vi "Pressure_control_TEMP.vi"(7 "Run Sequence":bool, 8 "user sequence, present (s) in, current step in, seq time in":T6, 9 "pressure parameters in":T1={"valve % open"=100.0, "Desired pressure"=0.0, "set Vapor sccm"=0.0, "set Gas sccm"=0.0, "Valve mode"=enum."% Open", "Pressure Mode"=enum."Abs. pressure", "analyte partial pressure"=100.0, "Turbo pump\nauto on"=TRUE} caption="Set pressure parameters" {"analyte partial pressure" min=0.0 max=100.0 step=5.0; "set Gas sccm" min=0 max=200 step=5; "set Vapor sccm" min=0 max=200 step=5; "Desired pressure" min=0.0 max=760.0 step=5.0; "valve % open" min=0.0 max=100.0 step=5.0 format="%#_2f"}, 10 "set temp":dbl, 11 "pressure control on? / DAQ IDs/errors in":T5) -> (0 "current step # out, shift register time out, seq button on?":T3, 1 "sequence over? USE THIS TO REINITIALIZE RUN SEQUENCE BUTTON SO PROGRAM ENDS":bool, 2 "save press/RH/gasflow/vaporflow - read valve position/pressure/vaporflow/gasflow":T2, 3 "pressure control on out, DAQ IDs/errors out":T4, 4 "sequence end date/time string":string, 5 "Temp setpoint":dbl)   [LabVIEW 2014]
uses:
  <vilib>/DAQmx/read.llb/DAQmx Read (Analog 1D DBL NChan 1Samp).vi
  <vilib>/DAQmx/write.llb/DAQmx Write (Analog 1D DBL NChan 1Samp).vi
  <vilib>/DAQmx/write.llb/DAQmx Write (Digital Bool 1Line 1Point).vi
panel:
  # "100%"
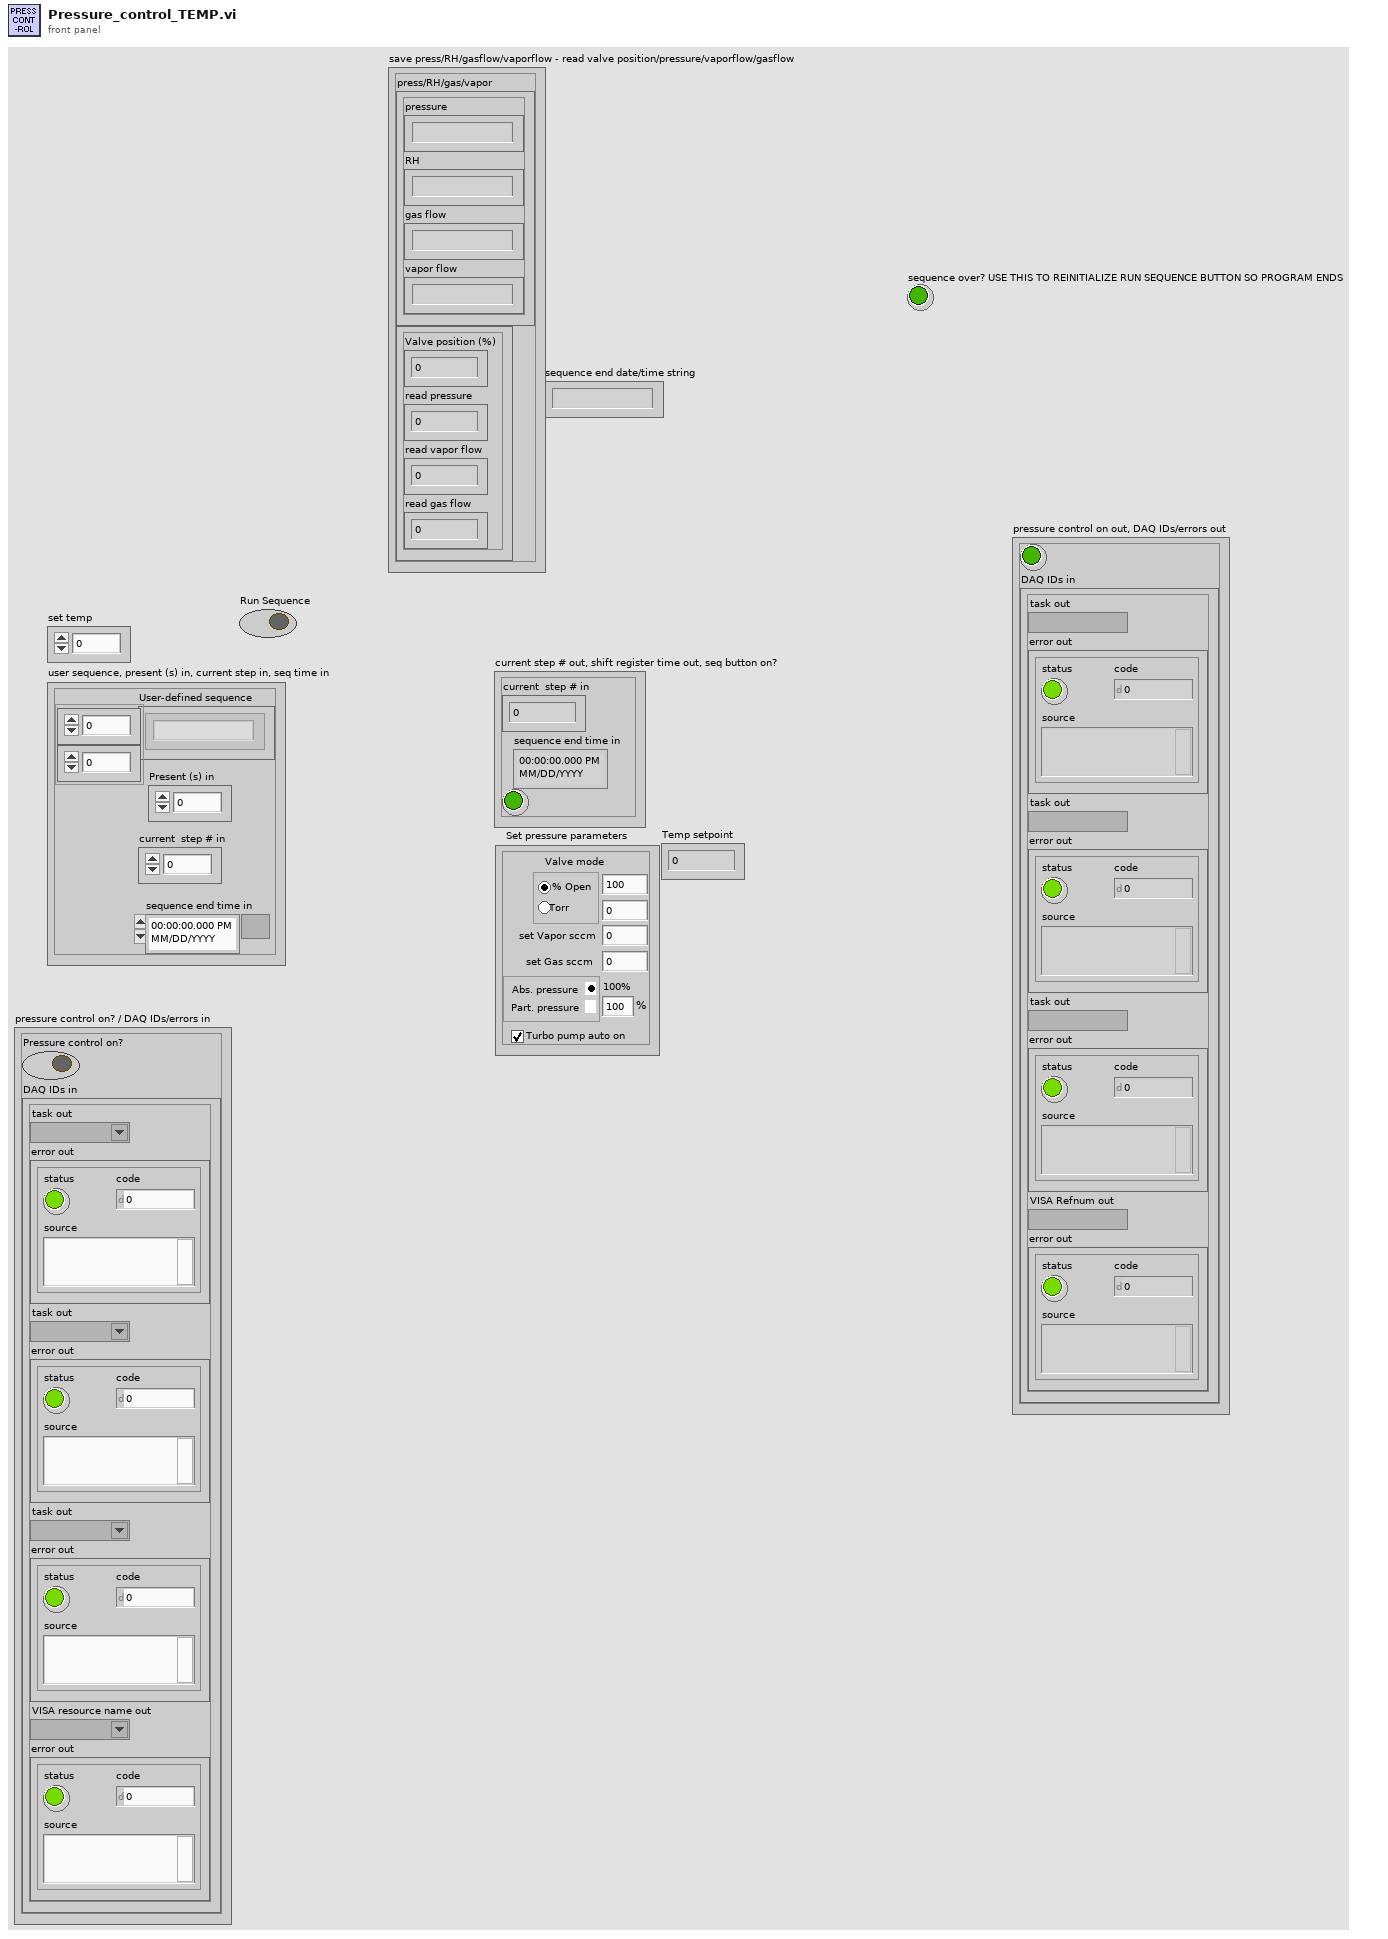
[diagram p1: front panel]
types:
  T1 = cluster{"valve % open":dbl, "Desired pressure":dbl, "set Vapor sccm":sgl, "set Gas sccm":sgl, "Valve mode":enum32{"% Open", "Torr "}, "Pressure Mode":enum32{"Abs. pressure", " Part. pressure"}, "analyte partial pressure":dbl, "Turbo pump\nauto on":bool}
  T2 = cluster{"press/RH/gas/vapor":cluster{"pressure":string, "RH":string, "gas flow":string, "vapor flow":string}, "Cluster":cluster{"Valve position (%)":dbl, "read pressure":dbl, "read vapor flow":dbl, "read gas flow":dbl}}
  T3 = cluster{"current  step # in":i32, "sequence end time in":timestamp, "Boolean":bool}
  T4 = cluster{"Boolean":bool, "DAQ IDs in":cluster{"task out":refnum<k21>, "error out":errorcluster, "task out":refnum<k21>, "error out":errorcluster, "task out":refnum<k21>, "error out":errorcluster, "VISA Refnum out":refnum<visa-resource-name>, "error out":errorcluster}}
  T5 = cluster{"Pressure control on?":bool, "DAQ IDs in":cluster{"task out":refnum<k21>, "error out":errorcluster, "task out":refnum<k21>, "error out":errorcluster, "task out":refnum<k21>, "error out":errorcluster, "VISA resource name out":refnum<visa-resource-name>, "error out":errorcluster}}
  T6 = cluster{"User-defined sequence":string[][], "Present (s) in":dbl, "current  step # in":i32, "sequence end time in":timestamp}
  T7 = cluster{"task out":refnum<k21>, "error out":errorcluster, "task out":refnum<k21>, "error out":errorcluster, "task out":refnum<k21>, "error out":errorcluster, "VISA resource name out":refnum<visa-resource-name>, "error out":errorcluster}
  T8 = cluster{"Valve position (%)":dbl, "pressure":dbl, "vapor flow":dbl, "gas flow":dbl}
  T9 = cluster{"pressure":string, "RH":string, "gas flow":string, "vapor flow":string}
  T10 = cluster{"String":dbl, "String":dbl, "Pressure Control":u32}
  T11 = cluster{"Valve position (%)":dbl, "read pressure":dbl, "read vapor flow":dbl, "read gas flow":dbl}
  T12 = cluster{"task out":refnum<k21>, "error out":errorcluster, "task out":refnum<k21>, "error out":errorcluster, "task out":refnum<k21>, "error out":errorcluster, "VISA Refnum out":refnum<visa-resource-name>, "error out":errorcluster}
  T13 = cluster{"press/RH/gas/vapor":cluster{"pressure":string, "RH":string, "gas flow":string, "vapor flow":string}, cluster{"Valve position (%)":dbl, "read pressure":dbl, "read vapor flow":dbl, "read gas flow":dbl}}
  T14 = cluster{"current  step # in":i32, "sequence end time in":timestamp, bool}
  T15 = cluster{bool, "DAQ IDs in":cluster{"task out":refnum<k21>, "error out":errorcluster, "task out":refnum<k21>, "error out":errorcluster, "task out":refnum<k21>, "error out":errorcluster, "VISA Refnum out":refnum<visa-resource-name>, "error out":errorcluster}}
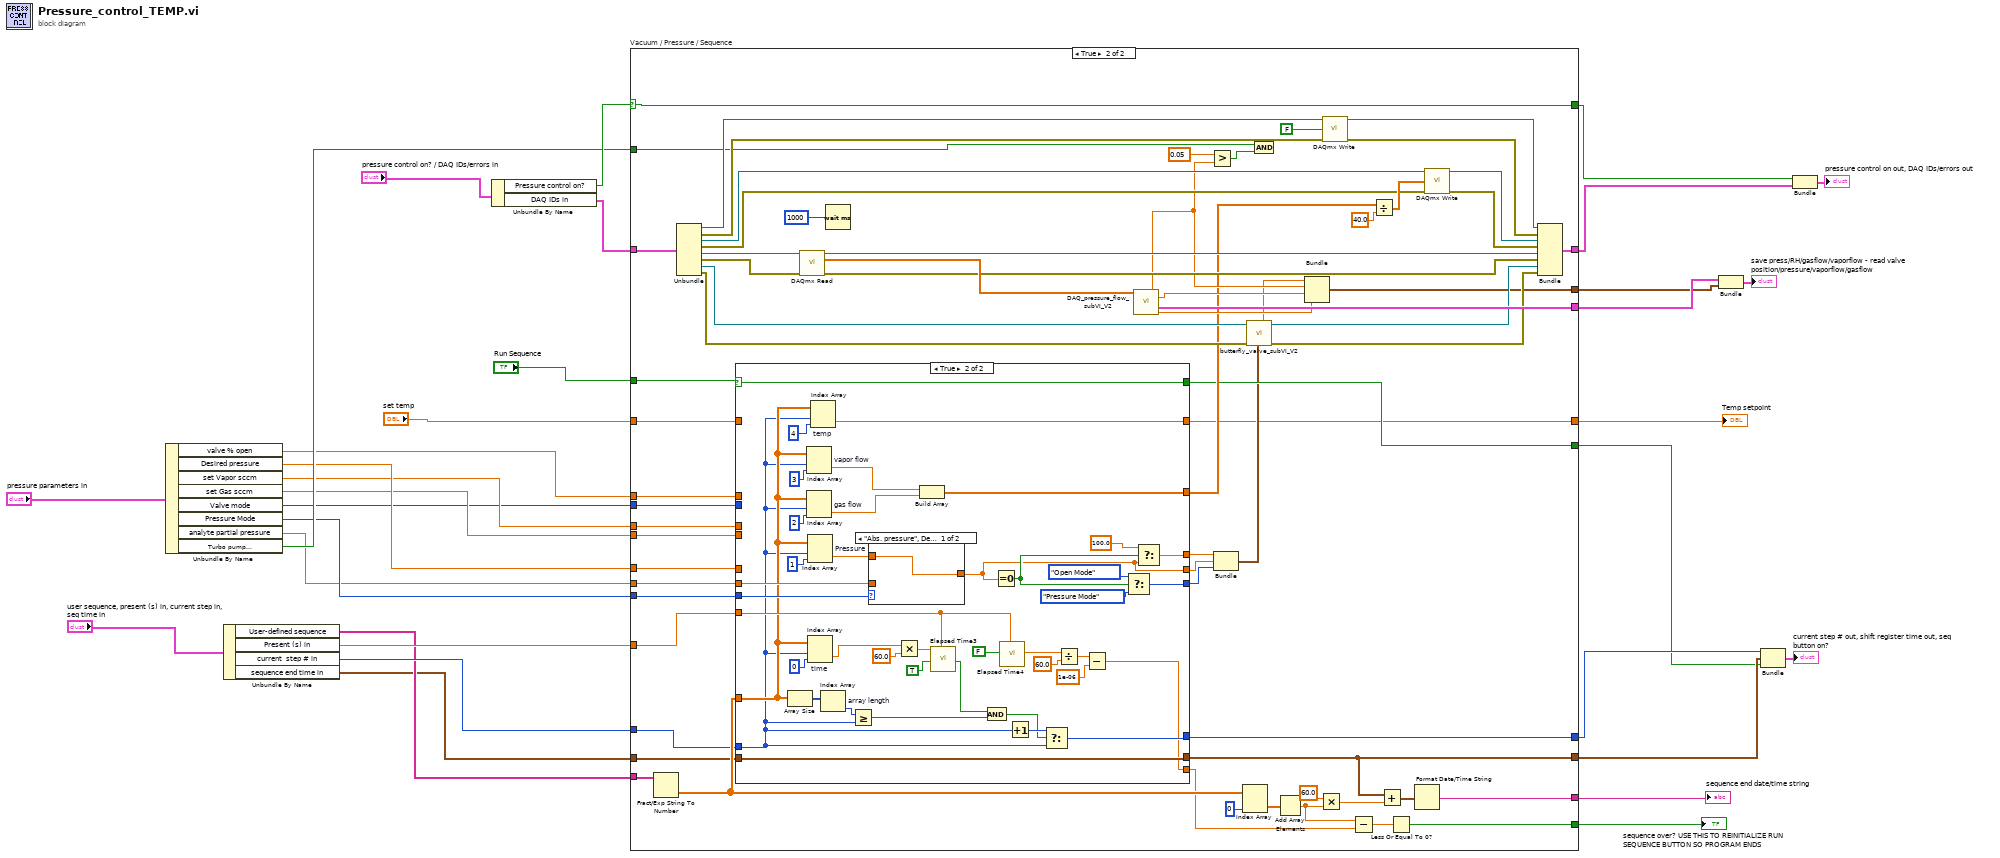
[diagram p0: block diagram]
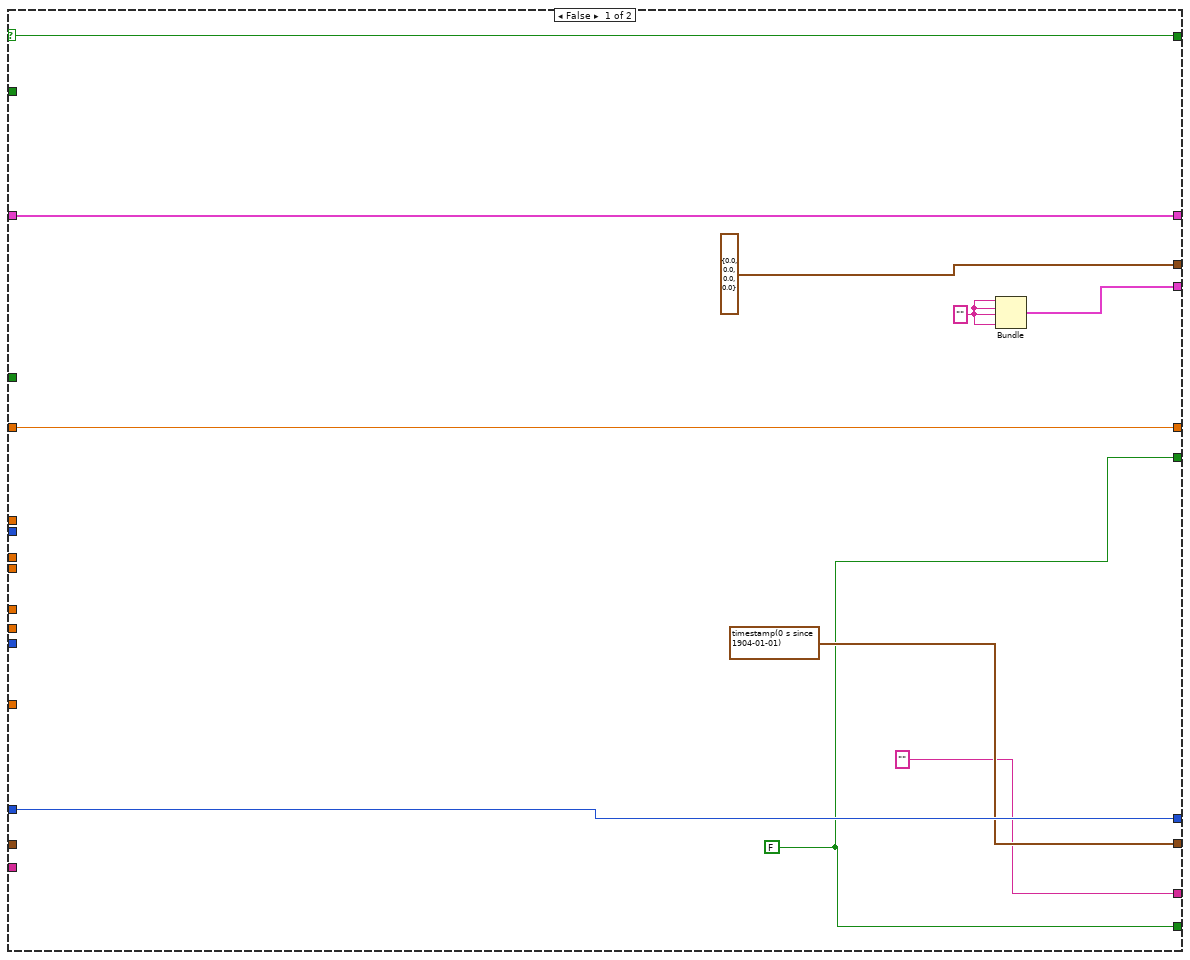
[diagram p2: hidden frame]
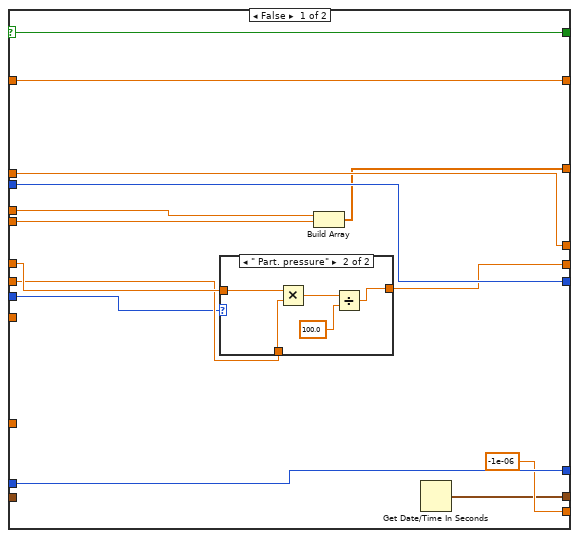
[diagram p3: hidden frame]
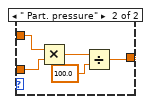
[diagram p5: hidden frame]
diagram:
  n1 = Unbundle By Name("pressure parameters in") -> ("valve % open"=w3:dbl, "Desired pressure"=w7:dbl, "set Vapor sccm"=w5:sgl, "set Gas sccm"=w6:sgl, "Valve mode"=w4:enum32{"% Open", "Torr "}, "Pressure Mode"=w9:enum32{"Abs. pressure", " Part. pressure"}, "analyte partial pressure"=w8:dbl, "Turbo pump\nauto on"=w10:bool)
  n2 = Unbundle By Name("user sequence, present (s) in, current step in, seq time in") -> ("User-defined sequence"=w26:string[][], "Present (s) in"=w27:dbl, "current  step # in"=w28:i32, "sequence end time in"=w25:timestamp)
  n3 = Unbundle By Name("pressure control on? / DAQ IDs/errors in") -> ("Pressure control on?"=w22:bool, "DAQ IDs in"=w23:T7)
  n4 = case "Vacuum / Pressure / Sequence" shown="True" w22 {
    selector: w22 -> [w34 w50]
    tunnel: w23 -> [w38 w104]
    tunnel: w28 -> [w42 w67]
    tunnel: [w42 w66] -> w18
    tunnel: [w35 w64] -> w16
    tunnel: [timestamp(0 s since 1904-01-01) ("seconds since 1Jan1904") w63] -> w17
    tunnel: [w40 w85] -> w14
    tunnel: [w38 w76] -> w20
    tunnel: w10 -> [_ w73]
    tunnel: w26 -> [_ w72]
    tunnel: ["" ("date/time string") w71] -> w32
    tunnel: [T8 {"Valve position (%)"=0.0, "pressure"=0.0, "vapor flow"=0.0, "gas flow"=0.0} w70] -> w13
    tunnel: w27 -> [_ w61]
    tunnel: "Run Sequence" -> [_ w60]
    tunnel: w25 -> [_ w59]
    tunnel: [w35 w58] -> w30
    tunnel: w7 -> [_ w57]
    tunnel: w3 -> [_ w56]
    tunnel: w5 -> [_ w55]
    tunnel: w9 -> [_ w54]
    tunnel: w4 -> [_ w53]
    tunnel: w6 -> [_ w52]
    tunnel: w8 -> [_ w51]
    tunnel: [w34 w50] -> w21
    tunnel: "set temp" -> [w33 w44]
    tunnel: [w33 w43] -> w2
    frame False {
      w35 = FALSE
      w39 = ""
      n5 = Bundle(w39, w39, w39, w39) -> (w40:cluster{string, string, string, string})  [unwired: 1 in]
    }
    frame True {
      n6 = Fract/Exp String To Number ("user sequence")(string=w72) -> (number=w68:dbl[][])  [unwired: 3 in, 1 out]
      n7 = Unbundle(w104) -> ("task out"=w97:refnum<k21>, "error out"=w96:errorcluster, "task out"=w98:refnum<k21>, "error out"=w99:errorcluster, "task out"=w100:refnum<k21>, "error out"=w101:errorcluster, "VISA resource name out"=w102:refnum<visa-resource-name>, "error out"=w103:errorcluster)
      n8 = case "Sequence" shown="True" w60 {
        selector: w60 -> [w119 w152]
        tunnel: w61 -> [_ w158]
        tunnel: [w122 w159] -> w66
        tunnel: w67 -> [w122 w130]
        tunnel: w52 -> [w117 _]
        tunnel: [w114 w136] -> w48
        tunnel: w68 -> [_ w131]
        tunnel: w53 -> [w121 _]
        tunnel: [w121 w137] -> w47
        tunnel: [-1e-06 w133] -> w62
        tunnel: [w119 w152] -> w64
        tunnel: [w118 w141] -> w49
        tunnel: w56 -> [w118 _]
        tunnel: [w116 w148] -> w65
        tunnel: [w115 w147] -> w63
        tunnel: w59 -> [_ w147]
        tunnel: w57 -> [w113 _]
        tunnel: w51 -> [w112 w145]
        tunnel: w54 -> [w111 w143]
        tunnel: w55 -> [w110 _]
        tunnel: [w109 w129] -> w43
        tunnel: w44 -> [w109 _]
        frame False {
          n9 = case shown="\" Part. pressure\"" w111 {
            tunnel: [w123 w124] -> w114
            tunnel: w113 -> [w123 w126]
            tunnel: w112 -> [_ w125]
            frame "Abs. pressure", Default {
            }
            frame " Part. pressure" {
              n10 = Multiply(x=w126, y=w125) -> (x*y=w128:dbl)
              n11 = Divide(x=w128, y=100.0 ("Analyte part. press. (%)")) -> (x/y=w124:dbl)
            }
          }
          n12 = Build Array(w110, w117) -> (w116:sgl[])
          n13 = Get Date/Time In Seconds() -> (seconds since 1Jan1904=w115:timestamp)
        }
        frame True {
          n14 = Array Size(array=w131) -> (size(s)=w169:i32[])
          n15 = Index Array "vapor flow"(array=w131, index (row)=w130, index (col)=3 ("disabled index (col)")) -> (element=w150:dbl)
          n16 = Index Array "gas flow"(array=w131, index (row)=w130, index (col)=2 ("disabled index (col)")) -> (element=w149:dbl)
          n17 = Index Array "Pressure"(array=w131, index (row)=w130, index (col)=1 ("disabled index (col)")) -> (element=w146:dbl)
          n18 = Index Array "time"(array=w131, index (row)=w130, index (col)=0) -> (element=w162:dbl)
          n19 = Index Array "temp"(array=w131, index (row)=w130, index (col)=4 ("disabled index (col)")) -> (element=w129:dbl)
          n20 = Index Array "array length"(array=w169) -> (element=w154:i32)  [unwired: 1 in]
          n21 = Greater Or Equal?(x=w154, y=w130) -> (x >= y?=w166:bool)
          n22 = case shown="\"Abs. pressure\", Default" w143 {
            tunnel: [w170 w171] -> w136
            tunnel: w146 -> [w170 w173]
            tunnel: w145 -> [_ w172]
            frame "Abs. pressure", Default {
            }
            frame " Part. pressure" {
              n23 = Multiply(x=w173, y=w172) -> (x*y=w174:dbl)
              n24 = Divide(x=w174, y=100.0 ("Analyte part. press. (%)")) -> (x/y=w171:dbl)
            }
          }
          n25 = Multiply(x=w162, y=60.0) -> (x*y=w153:dbl)
          n26 = Build Array(w150, w149) -> (w148:dbl[])
          n27 = call "Elapsed Time3"("Time Target (s)"=w153, "Auto Reset"=TRUE, "Set Start Time (s)"=w158) -> ("Time has Elapsed"=w144:bool)  [unwired: 9 in, 7 out]
          n28 = And(x=w144, y=w166) -> (x .and. y?=w151:bool)
          n29 = Equal To 0?(x=w136) -> (x = 0?=w140:bool)
          n30 = call "Elapsed Time4"("Reset"=FALSE, "Set Start Time (s)"=w158) -> ("Elapsed Time (s)"=w156:dbl)  [unwired: 10 in, 7 out]
          n31 = Increment(x=w130) -> (x+1=w160:i32)
          n32 = Select(t=w160, s=w151, f=w130) -> (s? t:f=w159:i32)
          n33 = Divide(x=w156, y=60.0) -> (x/y=w135:dbl)
          n34 = Subtract(x=w135, y=1e-06) -> (x-y=w133:dbl)
          n35 = Select(t=enum32{"Open Mode", "Pressure Mode"}."Open Mode" ("Pressure Control"), s=w140, f=enum32{"Open Mode", "Pressure Mode"}."Pressure Mode" ("Pressure Control")) -> (s? t:f=w137:enum32{"Open Mode", "Pressure Mode"})
          n36 = Select(t=100.0 ("valve % open 2"), s=w140, f=w136) -> (s? t:f=w141:dbl)
        }
      }
      n37 = call-poly <vilib>:"DAQmx Read.vi"("task/channels in"=w100, "error in"=w101) -> ("task out"=w80:refnum<k21>, "data"=w107:dbl[], "error out"=w79:errorcluster)  [unwired: 11 in]
      n38 = Wait (ms)(milliseconds to wait=u32 1000) -> ()  [unwired: 1 out]
      n39 = call "DAQ_pressure_flow_subVI_V2.vi"("vac press"=w107) -> ("read pressure"=w69:dbl, "read vapor flow"=w75:dbl, "press/RH/gas/vapor"=w85:T9, "read gas flow"=w74:dbl)  [unwired: 11 in]
      n40 = Greater?(x=0.05, y=w69) -> (0:w86:bool)
      n41 = Bundle("String"=w49, "String"=w48, "Pressure Control"=w47) -> (w45:T10)  [unwired: 1 in]
      n42 = Index Array(array=w68, index (col)=0 ("disabled index (col)")) -> (element=w94:dbl[])  [unwired: 1 in]
      n43 = call "butterfly_valve_subVI_V2.vi"("% open / desired pressure / pressure mode"=w45, "error in (no error)"=w103, "VISA Refnum in"=w102) -> ("error out"=w77:errorcluster, "VISA Refnum out"=w78:refnum<visa-resource-name>, "Valve position (%)"=w46:dbl)  [unwired: 6 in]
      n44 = And(x=w73, y=w86) -> ()  [unwired: 1 out]
      n45 = Add Array Elements(numeric array=w94) -> (sum=w88:dbl)
      n46 = Bundle("Valve position (%)"=w46, "read pressure"=w69, "read vapor flow"=w75, "read gas flow"=w74) -> (w70:T11)  [unwired: 1 in]
      n47 = Multiply(x=60.0 ("y"), y=w88) -> (x*y=w90:dbl)
      n48 = call-poly <vilib>:"DAQmx Write.vi"("task/channels in"=w97, "data"=FALSE, "error in"=w96) -> ("task out"=w84:refnum<k21>, "error out"=w83:errorcluster)  [unwired: 10 in, 1 out]
      n49 = Subtract(x=w88, y=w62) -> (x-y=w92:dbl)
      n50 = Divide(x=w65, y=40.0 ("Waveform")) -> (x/y=w106:dbl[])
      n51 = Add(x=w63, y=w90) -> (x+y=w89:timestamp)
      n52 = Less Or Equal To 0?(x=w92) -> (x <= 0?=w58:bool)
      n53 = Format Date/Time String(seconds (now)=w89) -> (date/time string=w71:string)  [unwired: 2 in]
      n54 = call-poly <vilib>:"DAQmx Write.vi"("task/channels in"=w98, "data"=w106, "error in"=w99) -> ("task out"=w82:refnum<k21>, "error out"=w81:errorcluster)  [unwired: 10 in, 1 out]
      n55 = Bundle("task out"=w84, "error out"=w83, "task out"=w82, "error out"=w81, "task out"=w80, "error out"=w79, "VISA Refnum out"=w78, "error out"=w77) -> (w76:T12)  [unwired: 1 in]
    }
  }
  "sequence end date/time string" <- w32
  "sequence over? USE THIS TO REINITIALIZE RUN SEQUENCE BUTTON SO PROGRAM ENDS" <- w30
  "Temp setpoint" <- w2
  n56 = Bundle("press/RH/gas/vapor"=w14, w13) -> (→"save press/RH/gasflow/vaporflow - read valve position/pressure/vaporflow/gasflow":T13)  [unwired: 1 in]
  n57 = Bundle("current  step # in"=w18, "sequence end time in"=w17, w16) -> (→"current step # out, shift register time out, seq button on?":T14)  [unwired: 1 in]
  n58 = Bundle(w21, "DAQ IDs in"=w20) -> (→"pressure control on out, DAQ IDs/errors out":T15)  [unwired: 1 in]
